vi "S4P to Sparameter.vi"(0 "S4P File Path":path=path "D:/TX.S4P", 1 "S4P Fomat":enum16{"RI", "dB"}(ring), 2 "Port Type":u16(ring), 4 "S-Parameter Name":T1(ring), 5 "nCmdShow":i16(ring) items=["SW_HIDE   ", "SW_SHOWNORMAL", "SW_SHOWMINIMIZED", "SW_SHOWMAXIMIZED", "SW_SHOWNOACTIVATE", "SW_SHOW", "SW_MINIMIZE", "SW_SHOWMINNOACTIVE", "SW_SHOWNA", "SW_RESTORE"]) -> (14 "Frequency(Hz)":dbl[](array[numeric]), 17 "Diff S-parameters Data":dbl[][](array[numeric]), 18 "TXT_Data":string, 19 "Single S-parameters Data":dbl[][](array[numeric]))   [LabVIEW 2011]
uses:
  subVI/logrecord/logrecordstring.vi
panel:
  out "Find?":bool
  out "Diff  S-Chart":dbl[][](graph)
  out "Single S-Chart":dbl[][](graph)
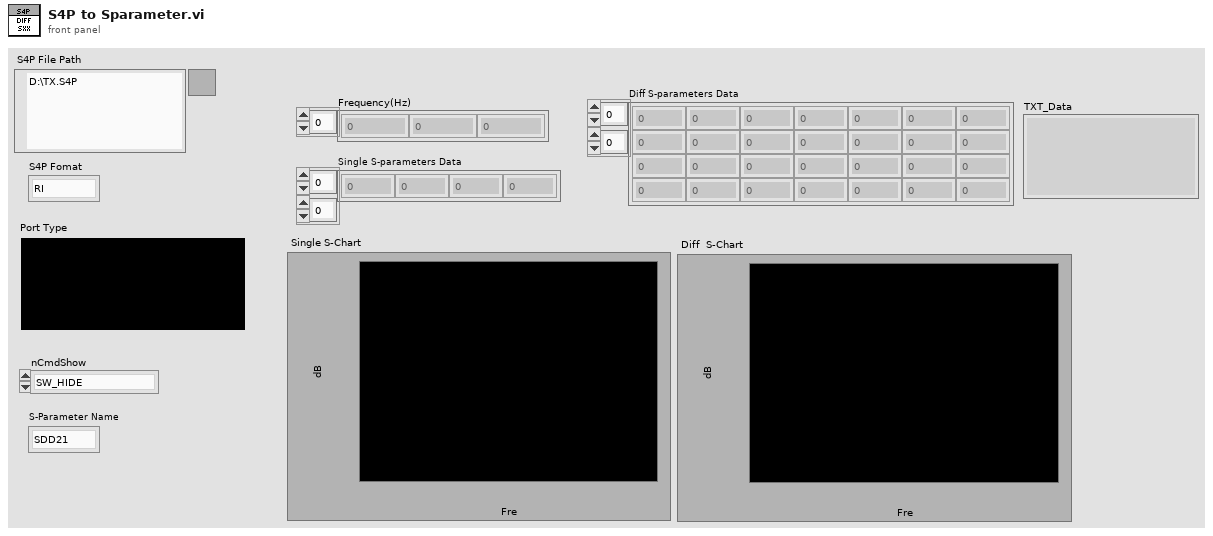
[diagram p1: front panel]
types:
  T1 = enum16{"SDD21", "SDD12", "SDD11", "SDD22", "SCD21", "SCD12", "SCD22", "SCD11", "SDC11", "SDC22", "SDC12", "SDC21", "SCC11", "SCC22", "SCC12", "SCC21"}
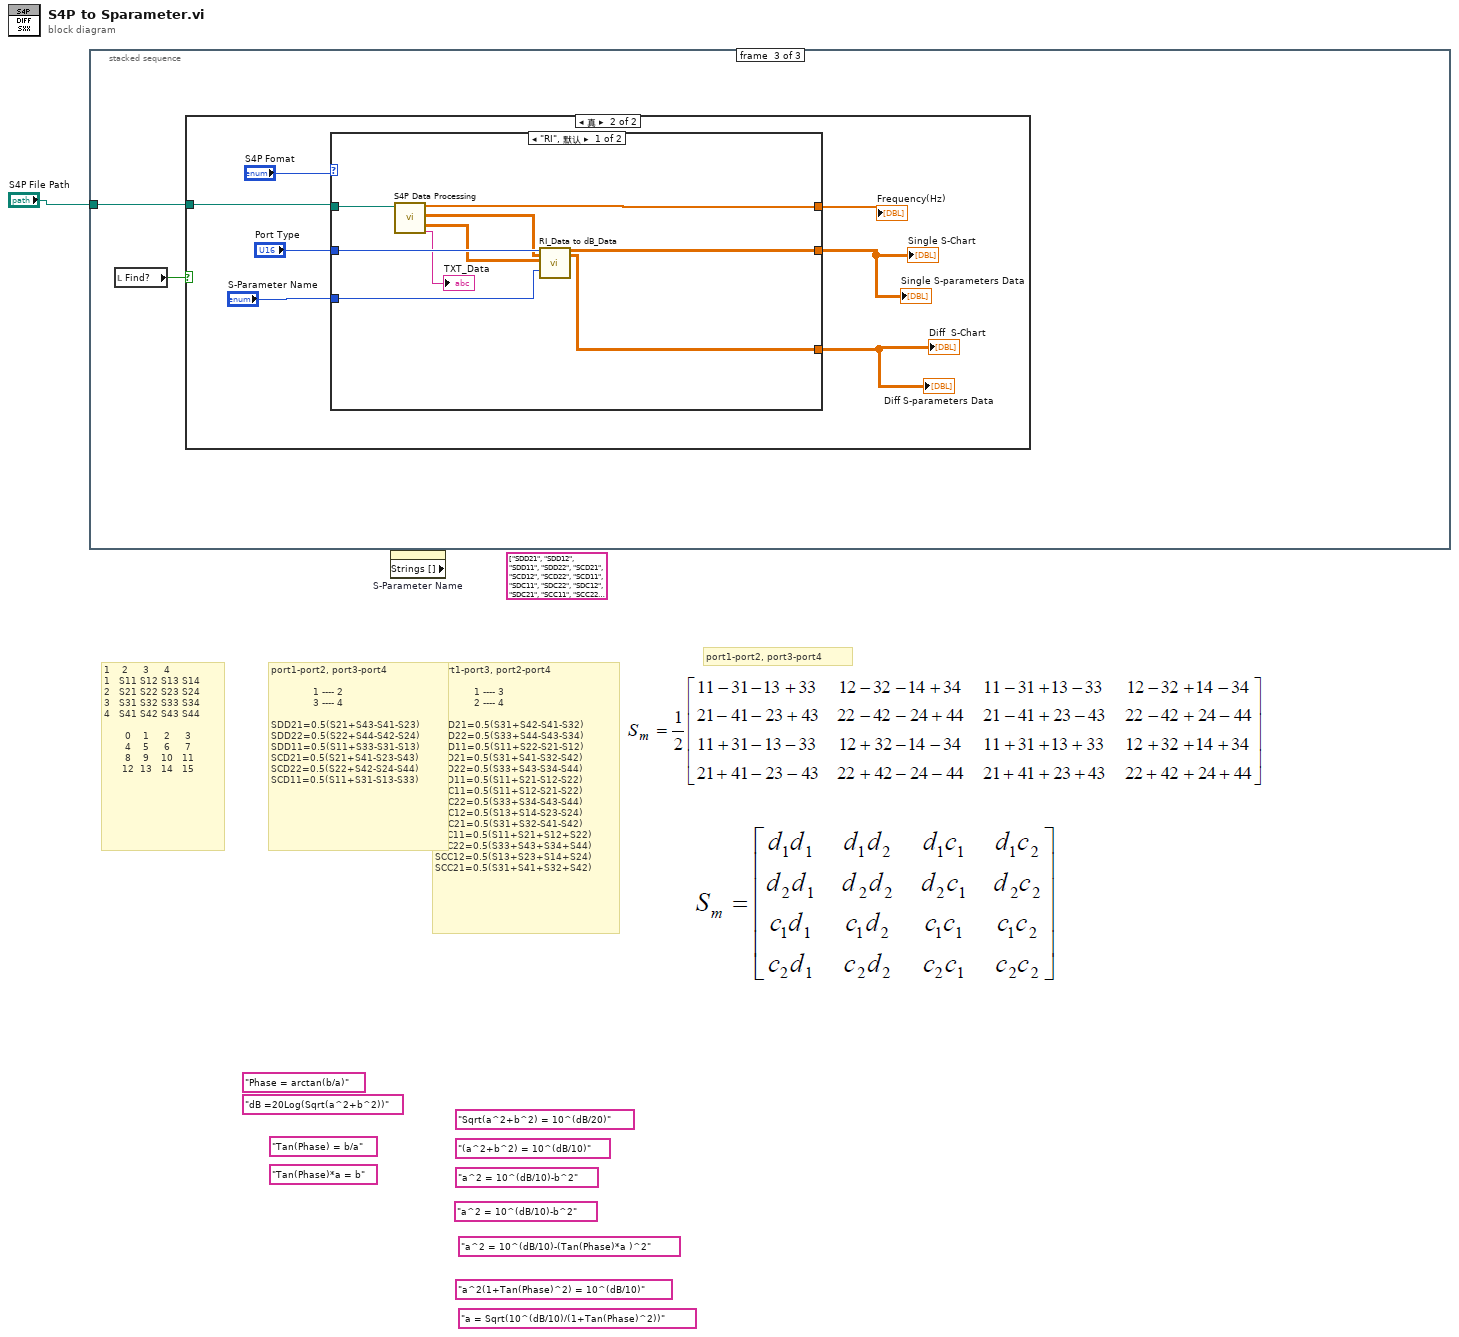
[diagram p0: block diagram]
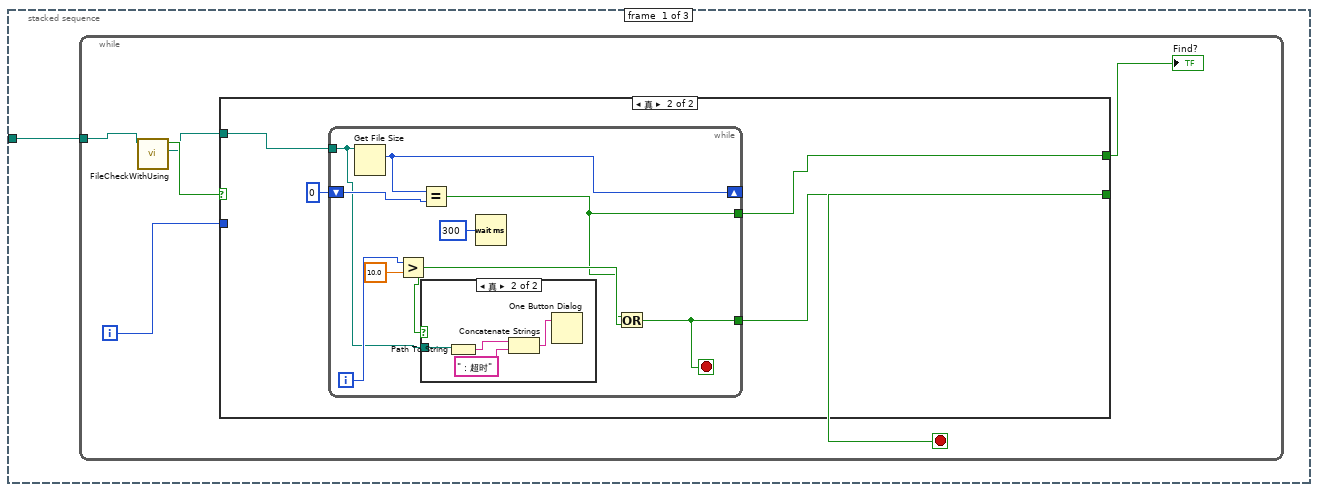
[diagram p2: hidden frame]
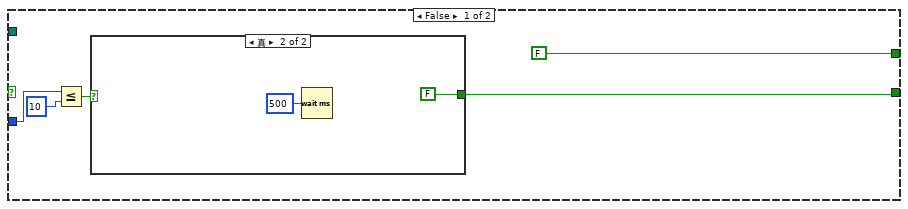
[diagram p3: hidden frame]
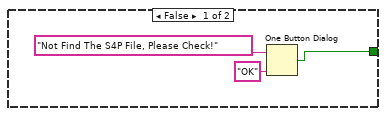
[diagram p4: hidden frame]
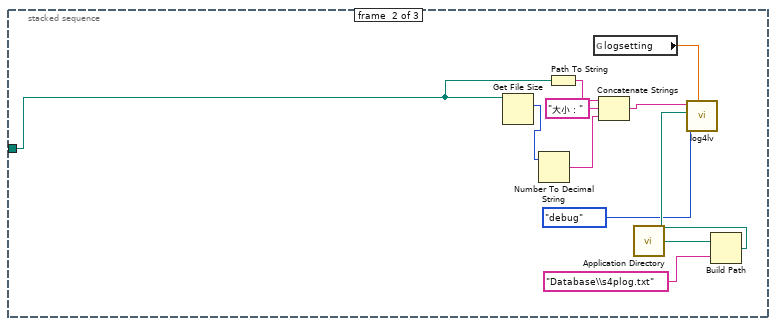
[diagram p6: hidden frame]
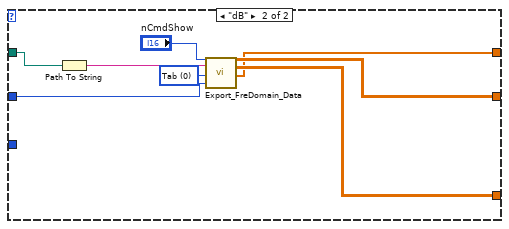
[diagram p8: hidden frame]
diagram:
  (unwired) string[] ["SDD21", "SDD12", "SDD11", "SDD22", "SCD21", "SCD12", "SCD22", "SCD11", "SDC11", "SDC22", "SDC12", "SDC21", "SCC11", "SCC22", "SCC12", "SCC21"] ("字符串[]")
  (unwired) "a = Sqrt(10^(dB/10)/(1+Tan(Phase)^2))"
  (unwired) "a^2(1+Tan(Phase)^2) = 10^(dB/10)"
  (unwired) "a^2 = 10^(dB/10)-(Tan(Phase)*a )^2"
  (unwired) "Tan(Phase)*a = b"
  (unwired) "a^2 = 10^(dB/10)-b^2"
  (unwired) "a^2 = 10^(dB/10)-b^2"
  (unwired) "(a^2+b^2) = 10^(dB/10)"
  (unwired) "Sqrt(a^2+b^2) = 10^(dB/20)"
  (unwired) "Tan(Phase) = b/a"
  (unwired) "dB =20Log(Sqrt(a^2+b^2))"
  (unwired) "Phase = arctan(b/a)"
  # "port1-port2, port3-port4"
  # "port1-port3, port2-port4\n \n             1 ---- 3\n             2 ---- 4\n\nSDD21=0.5(S31+S42-S41-S32)\nSDD22=0.5(S33+S44-S43-S34)\nSDD11=0.5(S11+S22-S21-S12)\nSCD21=0.5(S31+S41-S32-S42)\nSCD22=0.5(S33+S43-S34-S44)\nSCD11=0.5(S11+S21-S12-S22)\nSDC11=0.5(S11+S12-S21-S22)\nSDC22=0.5(S33+S34-S43-S44)\nSDC12=0.5(S13+S14-S23-S24)\nSDC21=0.5(S31+S32-S41-S42)\nSCC11=0.5(S11+S21+S12+S22)\nSCC22=0.5(S33+S43+S34+S44)\nSCC12=0.5(S13+S23+S14+S24)\nSCC21=0.5(S31+S41+S32+S42)"
  # "port1-port2, port3-port4\n\n              1 ---- 2\n              3 ---- 4\n\nSDD21=0.5(S21+S43-S41-S23)\nSDD22=0.5(S22+S44-S42-S24)\nSDD11=0.5(S11+S33-S31-S13)\nSCD21=0.5(S21+S41-S23-S43)\nSCD22=0.5(S22+S42-S24-S44)\nSCD11=0.5(S11+S31-S13-S33)"
  # "1    2     3     4\n1   S11 S12 S13 S14 \n2   S21 S22 S23 S24\n3   S31 S32 S33 S34\n4   S41 S42 S43 S44\n\n       0    1     2     3\n       4    5     6     7\n       8    9    10   11\n      12  13   14   15"
  n1 = stacked-sequence {
    tunnel: "S4P File Path" -> [w2 w41 w48]
    frame #0 {
      n2 = while {
        tunnel: w2 -> [w5]
        i -> [w7]
        stop <- w8 stop-if-true
        n3 = call "FileCheckWithUsing.vi"("路径"=w5) -> ("路径副本"=w3:path, "file exist"=w4:bool)  [unwired: 8 in, 1 out]
        n4 = case shown="真" w4 {
          tunnel: [w9 w19] -> w8
          tunnel: [FALSE w20] -> w6
          tunnel: w7 -> [w13 _]
          tunnel: w3 -> [_ w22]
          frame False {
            n5 = Less Or Equal?(x=w13, y=10) -> (x <= y?=w11:bool)
            n6 = case shown="真" w11 {
              tunnel: [w14 FALSE] -> w9
              frame False {
                n7 = One Button Dialog(message="Not Find The S4P File, Please Check!" ("消息"), button name ("OK")="OK" ("按钮名称（“确定”）")) -> (true=w14:bool)
              }
              frame True {
                n8 = Wait (ms)(milliseconds to wait=u32 500 ("等待时间（毫秒）")) -> ()  [unwired: 1 out]
              }
            }
          }
          frame True {
            n9 = while {
              tunnel: w22 -> [w25]
              shift-right: [w30] -> _
              shift-left: i64 0 ("size (in bytes)") -> [w29]
              tunnel: [w24] -> w20
              tunnel: [w23] -> w19
              i -> [w27]
              stop <- w23 stop-if-true
              n10 = Get File Size(file=w25) -> (size (in bytes)=w30:i64)  [unwired: 1 in, 2 out]
              n11 = Greater?(x=w27, y=10.0) -> (0:w26:bool)
              n12 = Equal?(x=w30, y=w29) -> (x = y?=w24:bool)
              n13 = case shown="真" w26 {
                tunnel: w25 -> [_ w35]
                frame False {
                }
                frame True {
                  n14 = Path To String(path=w35) -> (string=w33:string)
                  n15 = Concatenate Strings(w33, "：超时" ("字符串")) -> (w34:string)
                  n16 = One Button Dialog(message=w34) -> ()  [unwired: 1 in, 1 out]
                }
              }
              n17 = Wait (ms)(milliseconds to wait=u32 300 ("等待时间（毫秒）")) -> ()  [unwired: 1 out]
              n18 = Or(x=w24, y=w26) -> (x .or. y?=w23:bool)
            }
          }
        }
        "Find?" <- w6
      }
    }
    frame #1 {
      n19 = Get File Size(file=w41) -> (size (in bytes)=w44:i64)  [unwired: 1 in, 2 out]
      n20 = Number To Decimal String(number=w44) -> (decimal integer string=w43:string)  [unwired: 1 in]
      n21 = Path To String(path=w41) -> (string=w46:string)
      n22 = global read "全局.vi" "logsetting"() -> (w36:dbl)
      n23 = Concatenate Strings(w46, "大小：" ("字符串"), w43) -> (w42:string)
      n24 = call <vilib>:"Application Directory.vi"() -> ("Application Directory"=w40:path)
      n25 = Build Path(base path=w40, name or relative path="Database\\s4plog.txt" ("名称或相对路径")) -> (appended path=w38:path)
      n26 = call-poly "log4lv.vi"("logsetting"=w36, "logtype"=enum16{"error", "info", "debug"}."debug", "LogPath"=w38, "Msg"=w42) -> ()  [unwired: 7 in, 1 out]
    }
    frame #2 {
      n27 = local read "Find?"() -> (w47:bool)
      n28 = case shown="真" w47 {
        tunnel: w48 -> [_ w55]
        frame False {
        }
        frame True {
          n29 = case shown="\"RI\", 默认" "S4P Fomat" {
            tunnel: w55 -> [w64 w71]
            tunnel: [w63 w65] -> w53
            tunnel: "Port Type" -> [w62 w69]
            tunnel: "S-Parameter Name" -> [w61 _]
            tunnel: [w59 w67] -> w50
            tunnel: [w60 w66] -> w49
            frame "RI", Default {
              n30 = call "S4P Data Processing.vi"("S4P File Path"=w64) -> ("frequency(Hz)"=w63:dbl[], "Sxx_R"=w58:dbl[][], "Sxx_I"=w57:dbl[][], "TXT_Data"=→"TXT_Data":string)  [unwired: 15 in]
              n31 = call "RI_Data to dB_Data.vi"("Port Type"=w62, "Sxx_R"=w58, "Sxx_I"=w57, "S-Parameter Name"=w61) -> ("Single S-parameters Data"=w59:dbl[][], "Diff S-parameters Data"=w60:dbl[][])  [unwired: 14 in]
            }
            frame "dB" {
              w68 = i16 0 items=["Tab", "Comma"] ("delimiterType")
              n32 = Path To String(path=w71) -> (string=w70:string)
              n33 = call "Export_FreDomain_Data.vi"("nCmdShow"="nCmdShow", "szFileName"=w70, "delimiterType"=w68, "Port Type"=w69) -> ("Single S-parameters Data"=w67:dbl[][], "Diff S-parameters Data"=w66:dbl[][], "Frequency"=w65:dbl[])  [unwired: 20 in, 1 out]
            }
          }
          "Frequency(Hz)" <- w53
          "Single S-parameters Data" <- w50
          "Single S-Chart" <- w50
          "Diff S-parameters Data" <- w49
          "Diff  S-Chart" <- w49
        }
      }
    }
  }
  n34 = property on="S-Parameter Name" class="Enum (严格)" props=["Strings []"]() -> ()  [unwired: 2 in, 3 out]
